vi "OK.vi"(1 "布尔数组":bool[](array[boolean])) -> (0 "OK?":string)   [LabVIEW 2019]
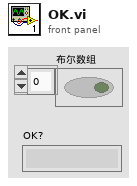
[diagram p1: front panel]
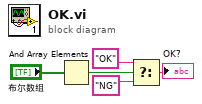
[diagram p0: block diagram]
diagram:
  n1 = And Array Elements(Boolean array="布尔数组") -> (logical AND=w4:bool)
  n2 = Select(t="OK", s=w4, f="NG") -> (s? t:f=→"OK?":string)
